vi "Constants.vi"() -> ()   [LabVIEW 2025, in "Runtime Configuration Support Inline Async Example Shared.lvlib"]
doc: "Use this Global VI to access the GUIDs assigned to the page resources of the Custom Device."
uses:
  Runtime Configuration Support Inline Async Example Shared.lvlib
panel:
  in  "Tab Control":enum32{"GUIDs", "Constants", "Properties"}(tab)
  in  "Runtime Configuration Support Inline Async Example":string="c91d0164-4b12-4160-bc5c-7f83ec49af3c"
  in  "Compiled.Settings":string="Compiled.Settings"
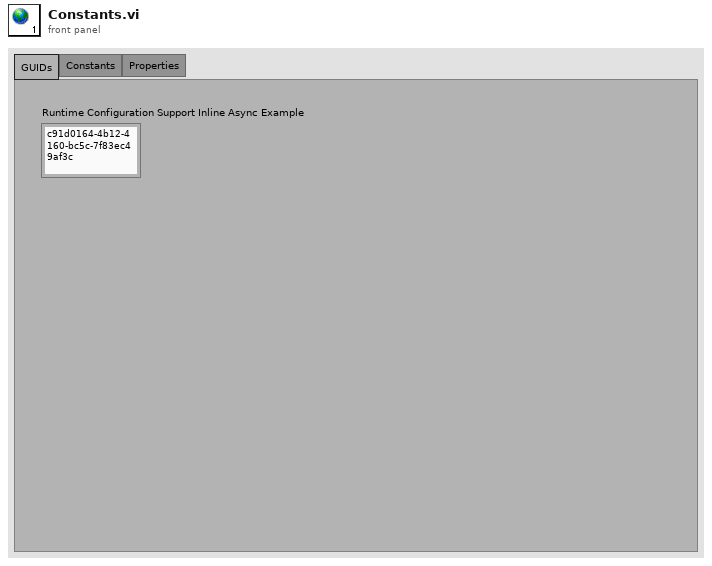
[diagram p1: front panel]
diagram:
